vi "4461 Delay Test.vi"() -> ()   [LabVIEW 2015]
uses:
  Utility VIs/Math VIs/FFT x(t) to dB,Degrees (1D).vi
  <vilib>/Analysis/NI_AALPro.lvlib
panel:
  out "Phase":T1(graph)
  out "Mag":T1(graph)
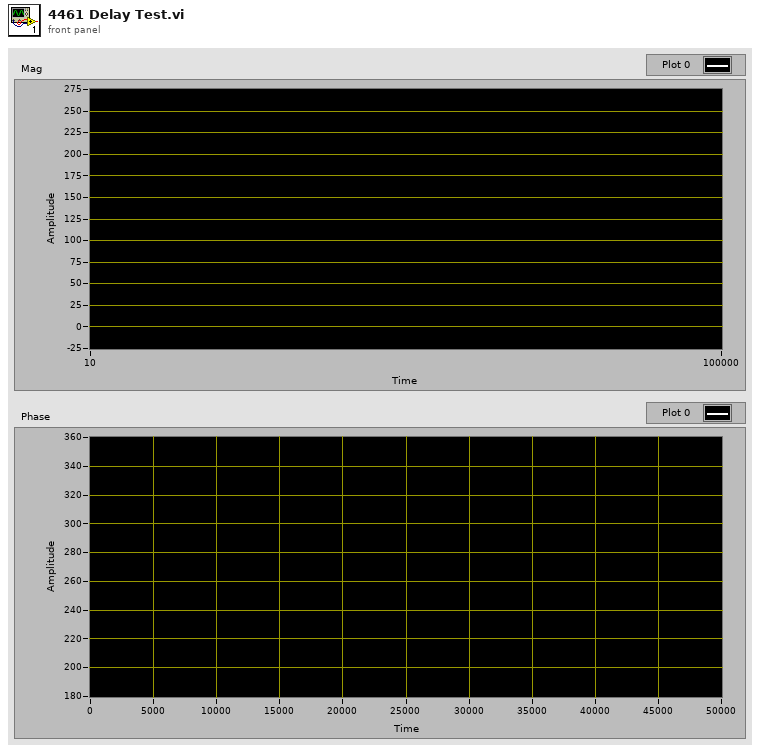
[diagram p1: front panel]
types:
  T1 = cluster{"Freq (Hz)":dbl[], "+Freq. Mag of FFT (dB rms)":dbl[]}
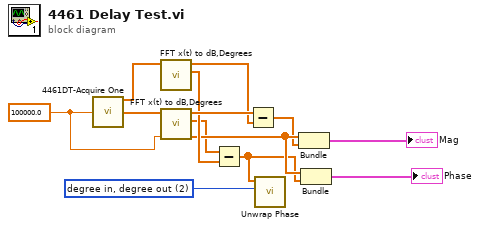
[diagram p0: block diagram]
diagram:
  w10 = 2 items=["radian in, radian out", "radian in, degree out", "degree in, degree out", "degree in, radian out"] ("phase unit")
  w12 = 100000.0 ("AI Fs")
  n1 = call "4461DT-Acquire One.vi"("AI Fs"=w12) -> ("Stimulus"=w9:dbl[], "Array"=w13:dbl[])  [unwired: 13 in]
  n2 = call-poly "FFT x(t) to dB,Degrees.vi"("X"=w9) -> ("+Freq Phase of FFT (degrees)"=w6:dbl[], "+Freq. Mag of FFT (dB rms)"=w7:dbl[])  [unwired: 8 in, 1 out]
  n3 = call-poly "FFT x(t) to dB,Degrees.vi"("Fs (Hz)"=w12, "X"=w13) -> ("Freq (Hz)"=w5:dbl[], "+Freq Phase of FFT (degrees)"=w3:dbl[], "+Freq. Mag of FFT (dB rms)"=w8:dbl[])  [unwired: 7 in]
  n4 = Subtract(x=w3, y=w6) -> (x-y=w2:dbl[])
  n5 = Subtract(x=w8, y=w7) -> (x-y=w4:dbl[])
  n6 = call <vilib>:"Unwrap Phase.vi"("phase unit"=w10, "Phase"=w2) -> ()  [unwired: 8 in, 2 out]
  n7 = Bundle("Freq (Hz)"=w5, w4) -> (→"Mag":cluster{"Freq (Hz)":dbl[], dbl[]})  [unwired: 1 in]
  n8 = Bundle("Freq (Hz)"=w5, w2) -> (→"Phase":cluster{"Freq (Hz)":dbl[], dbl[]})  [unwired: 1 in]
